vi "FlpLib ThreePhasePLL 0.vi"(0 "Vq":sgl, 1 "PLLgains":T3 {"proportional gain" step=0.125}, 2 "PLLrange":T2={"output high (Inf)"=inf, "output low (-Inf)"=0.0}, 3 "expectedFreq":sgl, 5 "dT":sgl, 9 "reset":bool, 11 "Phase In":sgl, 12 "PIstateIn":T1) -> (4 "gridFrequency":sgl, 14 "PIstateOut":T1, 15 "Phase Out":sgl)   [LabVIEW 2017]
uses:
  <vilib>/rvi/Analysis/control/PID/Typedef/niFpgaPID_PIGains.ctl
  <vilib>/rvi/Analysis/control/PID/Typedef/niFpgaPID_OutputRange.ctl
  <vilib>/rvi/Analysis/control/PID/Typedef/niFpgaPID_PIState.ctl
  <vilib>/rvi/Analysis/control/PID/Typedef/niFpgaPID_ManualControl.ctl
  Control/PI_Controller/FlpLib PI_Controller 0.vi
  <userlib>/_NI FLP Library/FPGA/outsideSCTL/FlpLib Multiply Shared Instance 0.vi
  <userlib>/_NI FLP Library/FPGA/outsideSCTL/FlpLib Add Shared Instance 0.vi
  <userlib>/_NI FLP Library/FPGA/outsideSCTL/FlpLib Subtract Shared Instance 0.vi
  <userlib>/_NI FLP Library/FPGA/outsideSCTL/FlpLib Greater Than Shared Instance 0.vi
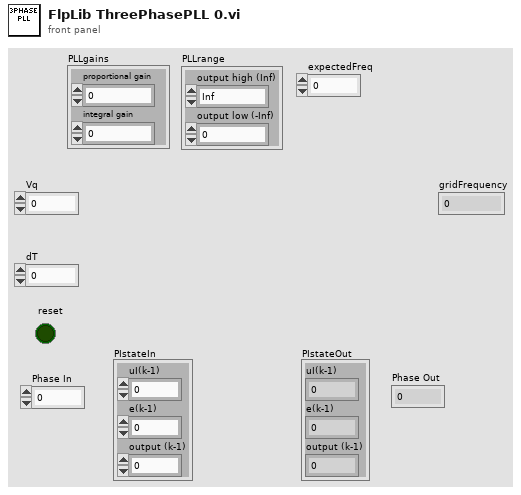
[diagram p1: front panel]
types:
  T1 = typedef "niFpgaPID_PIState.ctl" = cluster{"uI(k-1)":sgl, "e(k-1)":sgl, "output (k-1)":sgl}
  T2 = typedef "niFpgaPID_OutputRange.ctl" = cluster{"output high (Inf)":sgl, "output low (-Inf)":sgl}
  T3 = typedef "niFpgaPID_PIGains.ctl" = cluster{"proportional gain":sgl, "integral gain":sgl}
  T4 = typedef "niFpgaPID_ManualControl.ctl" = cluster{"manual? (F)":bool, "manual input (0)":sgl}
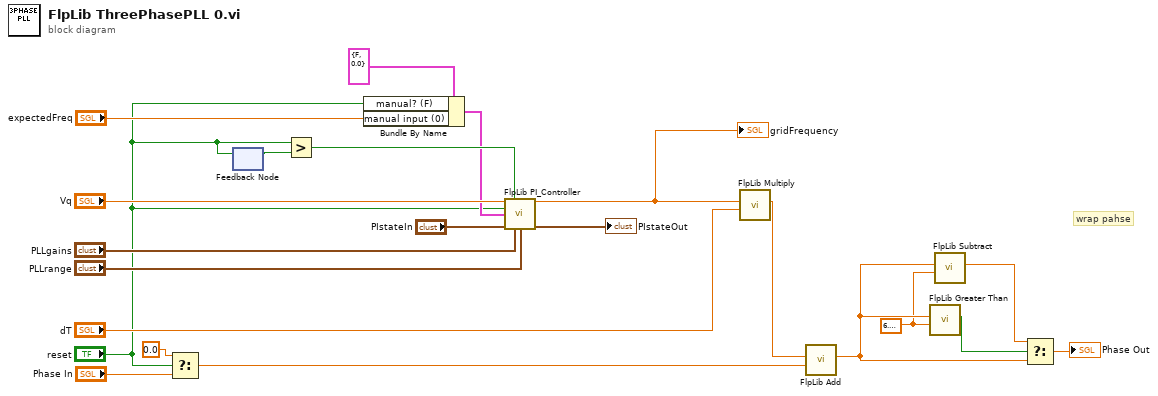
[diagram p0: block diagram]
diagram:
  w9 = sgl 6.2831855
  # "wrap pahse"
  n1 = Select(t=sgl 0.0, s="reset", f="Phase In") -> (s? t:f=w15:sgl)
  n2 = feedback-in #1("reset") -> ()
  n3 = feedback #1() -> (w6:bool)  [unwired: 1 in]
  n4 = Greater?(x="reset", y=w6) -> (0:w5:bool)
  n5 = Bundle By Name(cluster=T4 {"manual? (F)"=FALSE, "manual input (0)"=0.0} ("manual control"), "manual? (F)"="reset", "manual input (0)"="expectedFreq") -> (w3:T4)
  n6 = call-poly "FlpLib PI_Controller.vi"("error"="Vq", "reset? (F)"=w5, "enable bumpless transfer? (F)"="reset", "manual control"=w3, "state in"="PIstateIn", "gains"="PLLgains", "output range"="PLLrange") -> ("output"=w8:sgl, "state out"=→"PIstateOut":T1)  [unwired: 5 in, 2 out]
  "gridFrequency" <- w8
  n7 = call-poly <userlib>:"FlpLib Multiply.vi"("y"="dT", "x"=w8) -> ("x*y"=w16:sgl)  [unwired: 5 in]
  n8 = call-poly <userlib>:"FlpLib Add.vi"("y"=w15, "x"=w16) -> ("x+y"=w14:sgl)  [unwired: 5 in]
  n9 = call-poly <userlib>:"FlpLib Greater Than.vi"("y"=w9, "x"=w14) -> ("x > y?"=w19:bool)  [unwired: 5 in]
  n10 = call-poly <userlib>:"FlpLib Subtract.vi"("y"=w9, "x"=w14) -> ("x-y"=w13:sgl)  [unwired: 5 in]
  n11 = Select(t=w13, s=w19, f=w14) -> (s? t:f=→"Phase Out":sgl)
